vi "save snapshot.vi"(8 "error in (no error)":errorcluster, 11 "data directory":path) -> (0 "error out":errorcluster)   [LabVIEW 2017]
uses:
  popup panels/control panel globals.vi
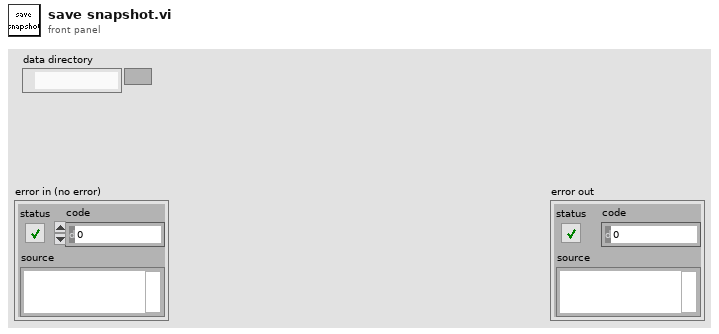
[diagram p1: front panel]
types:
  T1 = typedef "imagedata.ctl" = cluster{"image type":i32, "image depth":i32, "image":u8[], "mask":u8[], "colors":u32[], "Rectangle":cluster{"left":i16, "top":i16, "right":i16, "bottom":i16}}
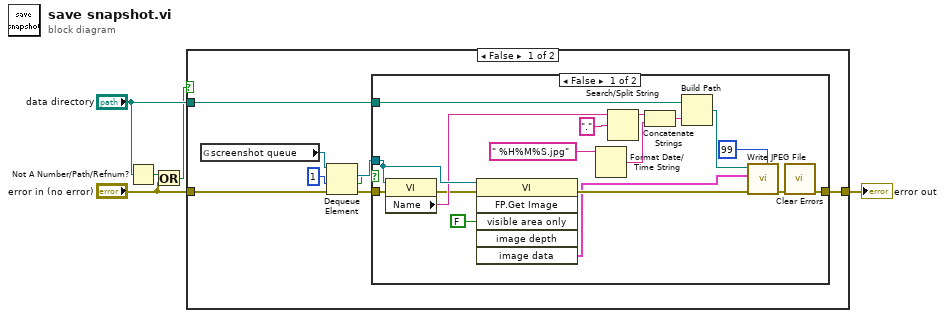
[diagram p0: block diagram]
diagram:
  n1 = Not A Number/Path/Refnum?(number/path/refnum="data directory") -> (NaN/Path/Refnum?=w4:bool)
  n2 = Or(x=w4, y="error in (no error)") -> (x .or. y?=w2:bool)
  n3 = case shown="False" w2 {
    tunnel: "data directory" -> [w8 _]
    tunnel: "error in (no error)" -> [w7 w32]
    tunnel: [w6 w32] -> w1
    frame False {
      n4 = global read "control panel globals.vi" "screenshot queue"() -> (w13:refnum<queue>)
      n5 = Dequeue Element(queue=w13, timeout in ms (-1)=1, error in (no error)=w7) -> (element=w11:refnum<vi>, timed out?=w9:bool, error out=w10:errorcluster)  [unwired: 1 out]
      n6 = case shown="False" w9 {
        tunnel: w11 -> [w24 _]
        tunnel: w10 -> [w18 w31]
        tunnel: [w15 w31] -> w6
        tunnel: w8 -> [w14 _]
        frame False {
          n7 = property class="VI"(reference=w24, error in=w18) -> (error out=w17:errorcluster, "Name"=w23:string)  [unwired: 1 out]
          n8 = invoke class="VI" method="FP.Get Image"(reference=w24, error in=w17, "visible area only"=FALSE ("Visible Area Only")) -> (error out=w28:errorcluster, "image data"=w27:T1)  [unwired: 3 in, 4 out]
          n9 = Format Date/Time String(time format string (%c)=" %H%M%S.jpg") -> (date/time string=w19:string)  [unwired: 2 in]
          n10 = Search/Split String(string=w23, search string/char (-)=".") -> (substring before match=w21:string)  [unwired: 1 in, 2 out]
          n11 = Concatenate Strings(w21, w19) -> (w29:string)
          n12 = Build Path(base path=w14, name or relative path=w29) -> (appended path=w30:path)
          n13 = call <vilib>:"Write JPEG File.vi"("quality (80)"=99, "error in (no error)"=w28, "image data"=w27, "path to JPEG file"=w30) -> ("error out"=w16:errorcluster)  [unwired: 6 in, 1 out]
          n14 = call <vilib>:"Clear Errors.vi"("error in (no error)"=w16) -> ("error out"=w15:errorcluster)  [unwired: 5 in, 1 out]
        }
        frame True {
        }
      }
    }
    frame True {
    }
  }
  "error out" <- w1
